vi "high_pass_filter_selector.vi"(0 "Signal input":dbl, 7 "Order":enum16{"1st order", "2nd order", "3rd order"}(ring), 11 "High pass":bool, 13 "Corner period":dbl(slide)=30.0 scale=1.0..1000.0) -> (8 "Signal output":dbl format="%.2f")   [LabVIEW 2016]
doc: "Use this VI to select the order of high pass filter. If High pass button is pushed the Signal input will be filtered, otherwise , the Signal input will be the same.\n\nInputs:\nSignal input,\nOrder,\nHigh pass,\nCorner period.\nOutputs:\nSignal output.\n\nMuhannad Alghamdi\nCSUSB Physics 350"
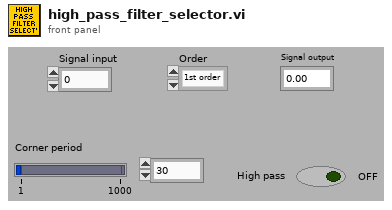
[diagram p1: front panel]
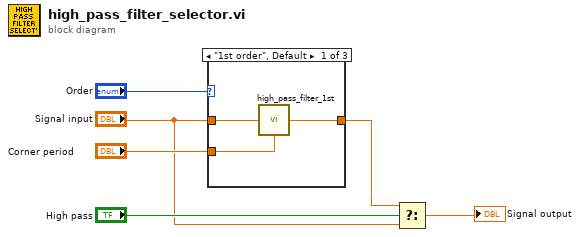
[diagram p0: block diagram]
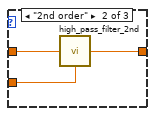
[diagram p2: hidden frame]
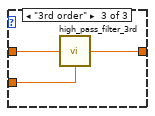
[diagram p3: hidden frame]
diagram:
  n1 = case shown="\"1st order\", Default" "Order" {
    tunnel: "Signal input" -> [w9 w12 w15]
    tunnel: "Corner period" -> [w8 w11 w14]
    tunnel: [w7 w10 w13] -> w2
    frame "1st order", Default {
      n2 = call "high_pass_filter_1st.vi"("Input"=w9, "Corner period"=w8) -> ("Output"=w7:dbl)  [unwired: 13 in]
    }
    frame "2nd order" {
      n3 = call "high_pass_filter_2nd.vi"("Input"=w12, "Corner period"=w11) -> ("Output"=w10:dbl)  [unwired: 13 in]
    }
    frame "3rd order" {
      n4 = call "high_pass_filter_3rd.vi"("Input"=w15, "Corner period"=w14) -> ("Output"=w13:dbl)  [unwired: 13 in]
    }
  }
  n5 = Select(t=w2, s="High pass", f="Signal input") -> (s? t:f=→"Signal output":dbl)
